vi "No File Loaded Message.vi"() -> (0 "no file loaded string":string)   [LabVIEW 2021, in "DSF Core.lvlib"]
uses:
  DSF Core.lvlib
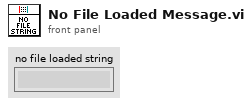
[diagram p1: front panel]
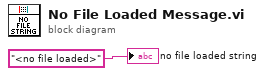
[diagram p0: block diagram]
diagram:
  "no file loaded string" <- "<no file loaded>" ("Front Panel Window:Title")
